vi "Write unit ID.vi"(8 "error in (no error)":errorcluster, 10 "unit ID":u8=1, 11 "Modbus Slave configuration in":refnum<class "Modbus Slave configuration.lvclass">) -> (0 "error out":errorcluster, 3 "Modbus Slave configuration out":refnum<class "Modbus Slave configuration.lvclass">)   [LabVIEW 2013, in "Modbus Slave configuration.lvclass"]
uses:
  Modbus Slave configuration.lvclass
  Modbus Slave configuration.lvclass/Modbus Slave configuration.ctl
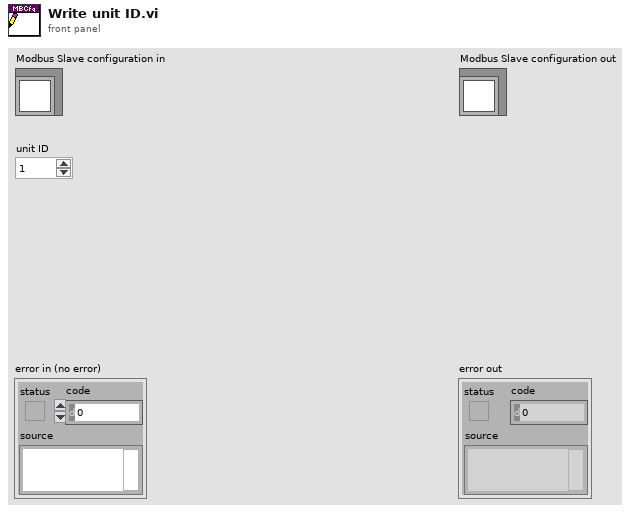
[diagram p1: front panel]
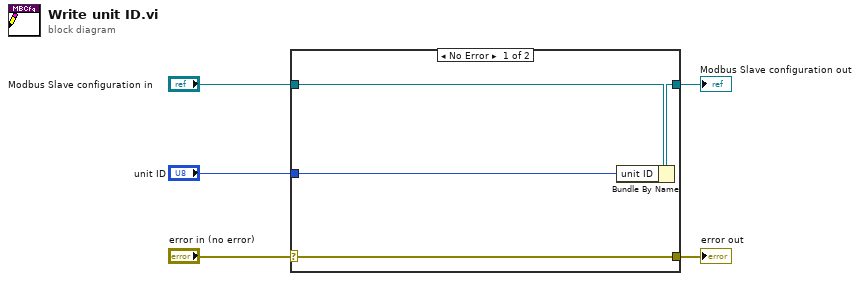
[diagram p0: block diagram]
diagram:
  n1 = case shown="No Error" "error in (no error)" {
    selector: "error in (no error)" -> [w9 w10]
    tunnel: [w9 w10] -> w4
    tunnel: [w7 w11] -> w2
    tunnel: "Modbus Slave configuration in" -> [w8 w11]
    tunnel: "unit ID" -> [w6 _]
    frame No Error {
      n2 = Bundle By Name(cluster=w8, "unit ID"=w6) -> (w7:refnum<class "Modbus Slave configuration.lvclass">)
    }
    frame Error {
    }
  }
  "error out" <- w4
  "Modbus Slave configuration out" <- w2
